vi "xmlParse.vi"() -> ()   [LabVIEW 2018]
doc: "This example demonstrates how to query an XML document by using an XPath expression and returns all the nodes that match the XPath expression."
uses:
  <vilib>/xml/Close Reference(Node).vi
  <resource>/objmgr/DOMUserDefRef.rc
  <vilib>/xml/NI_XML.lvlib
panel:
  out "concatenated string":string
  out "Array":string[](array[string])
  out "offset past replacement 2":i32
  out "result string 2":string
  out "substring before match 2":string
  out "offset past replacement":i32
  in  "Numeric":i32
  out "size(s)":i32
  out "result string":string
  out "element":string
  in  "XML File Path":path=path "C:/LabviewFiles/LabView/learning(Lee)/LVU examples/xmlParsing/ETNT22116.xml"
  out "XML":string
  in  "XPath Expression":string
  out "Search Results":string[](array[string])
  # "filter for software"
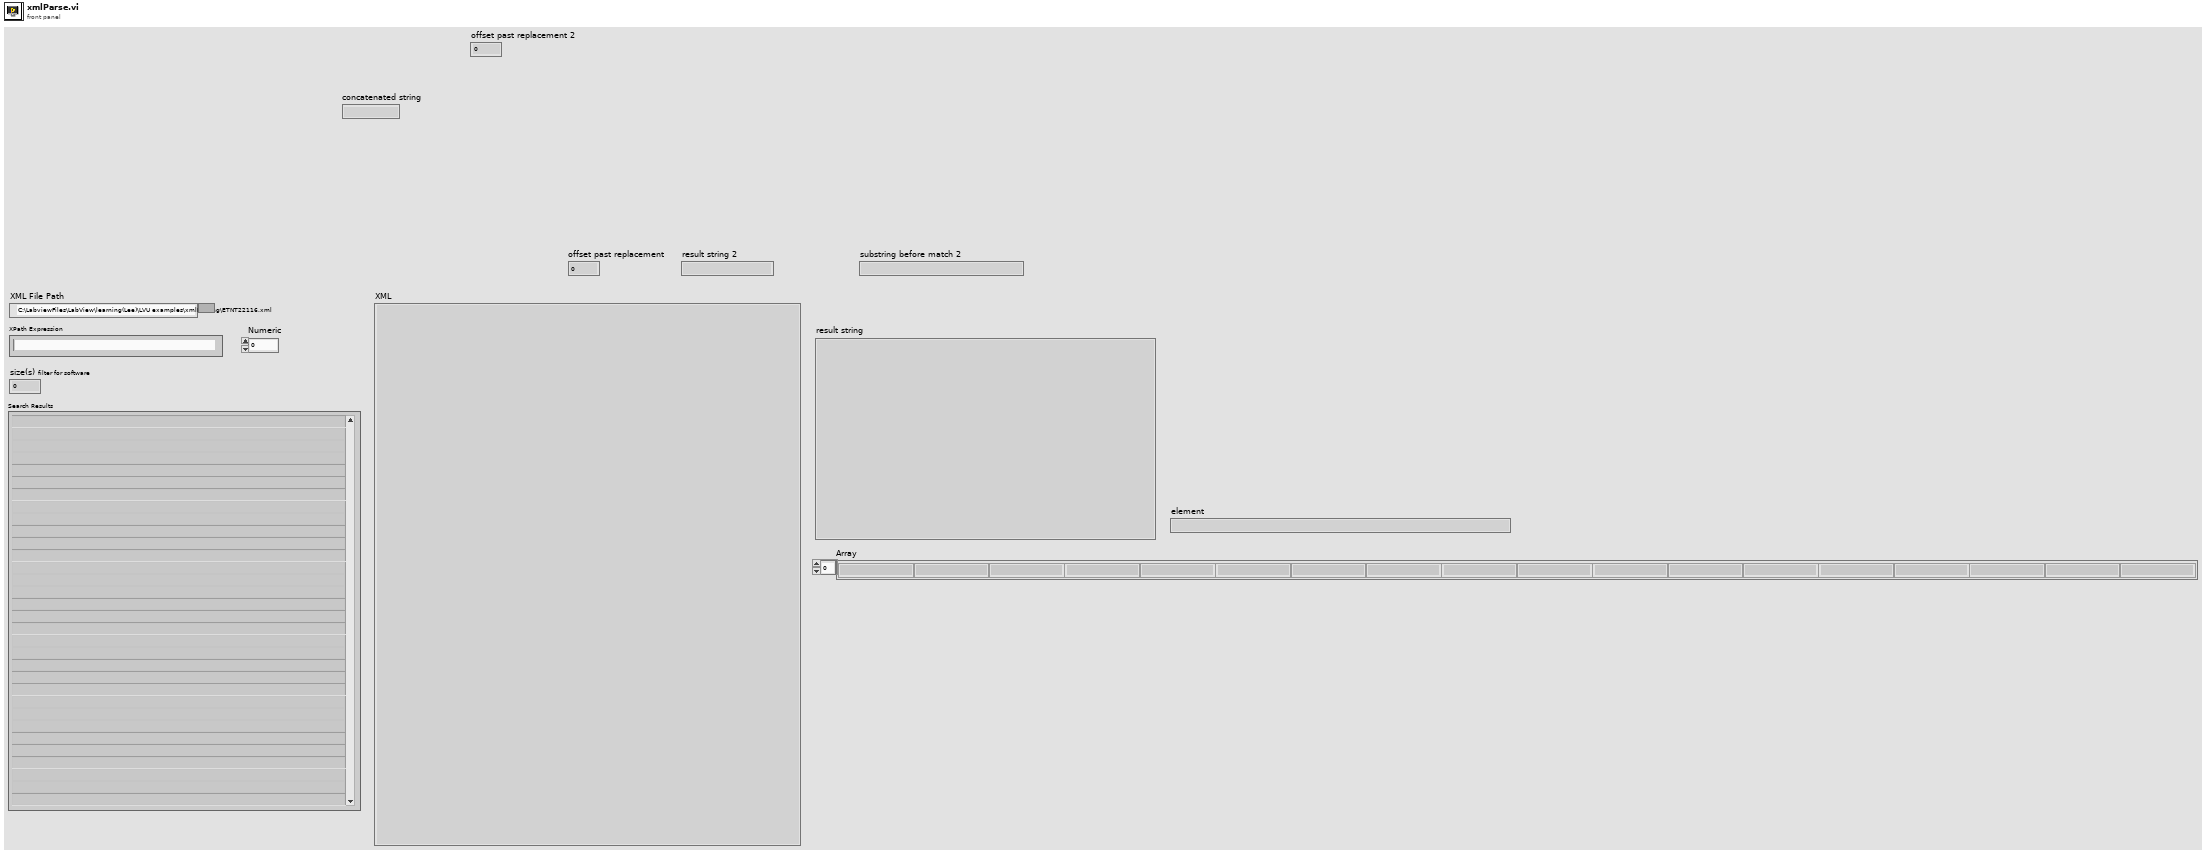
[diagram p1: front panel]
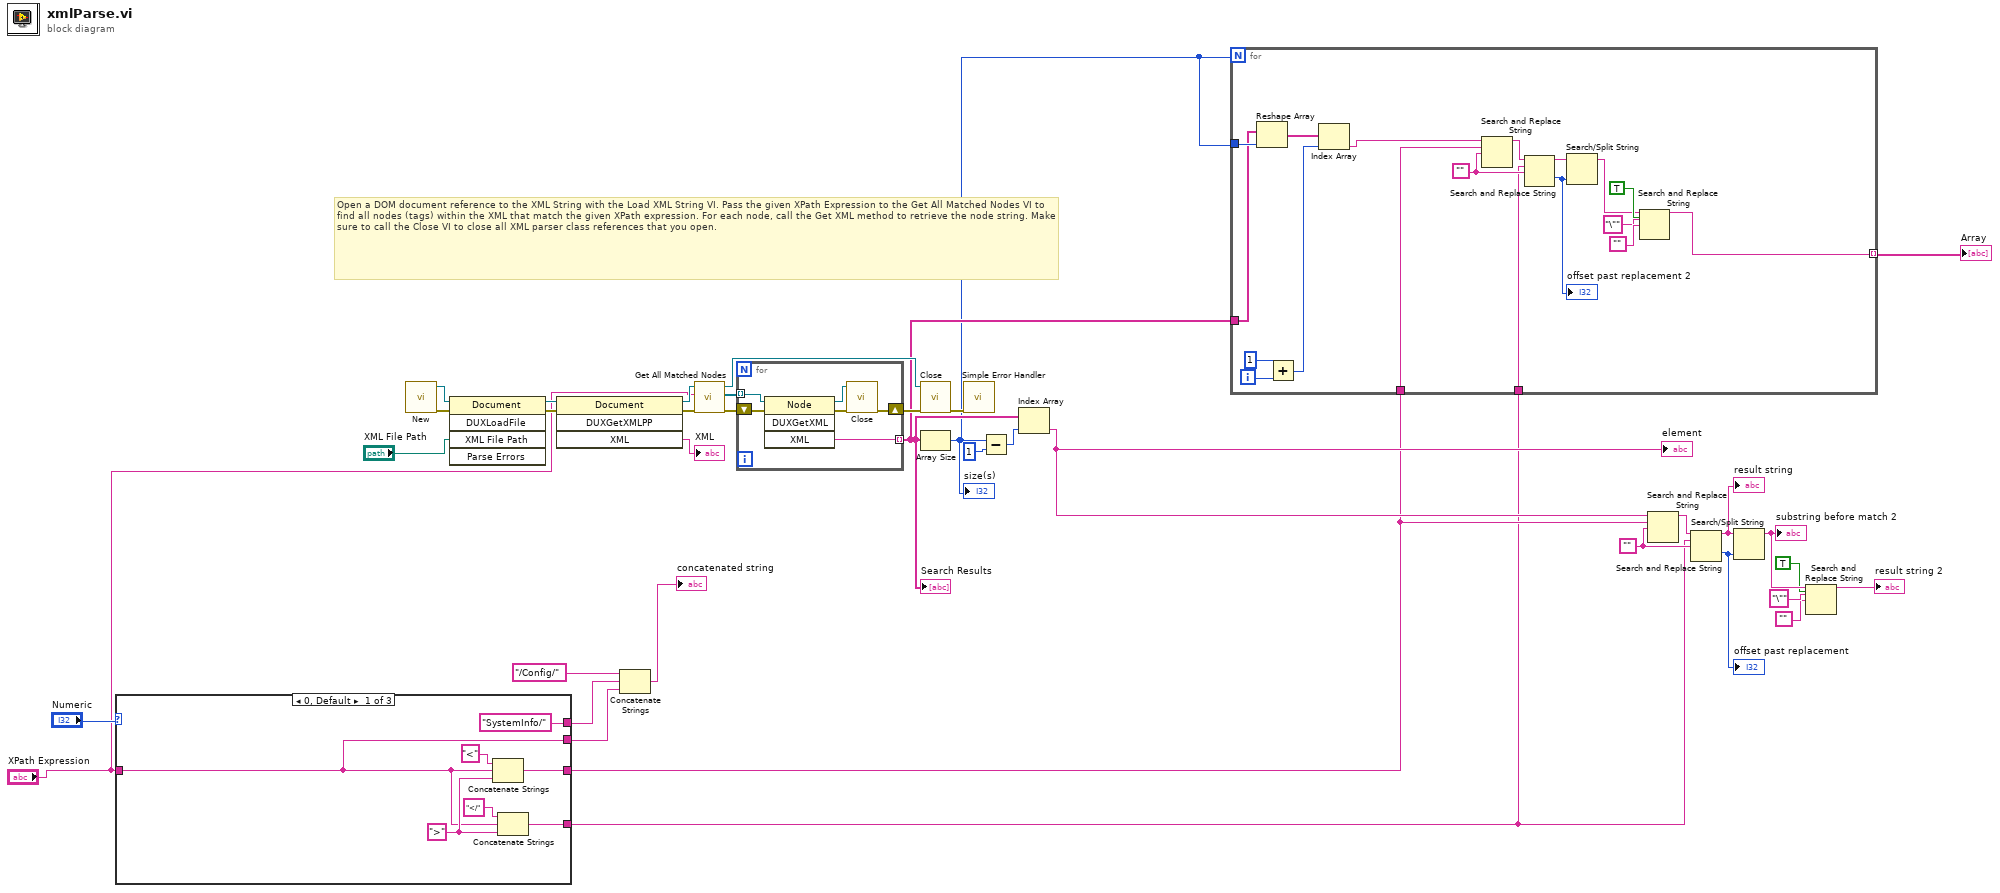
[diagram p0: block diagram]
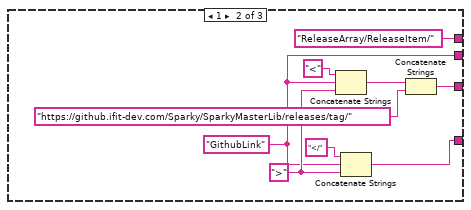
[diagram p2: hidden frame]
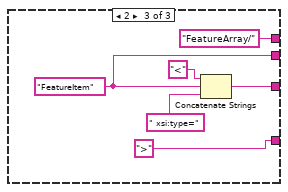
[diagram p3: hidden frame]
diagram:
  w15 = ""
  # "Open a DOM document reference to the XML String with the Load XML String VI. Pass the given XPath Expression to the Get All Matched Nodes VI to find all nodes (tags) within the XML that match the given XPath expression. For each node, call the Get XML method to retrieve the node string. Make sure to call the Close VI to close all XML parser class references that you open."
  n1 = case shown="0, Default" "Numeric" {
    tunnel: ["SystemInfo/" "ReleaseArray/ReleaseItem/" "FeatureArray/"] -> w18
    tunnel: [w39 w48 ">" ("string")] -> w4
    tunnel: [w38 w47 w56] -> w5
    tunnel: [w37 w44 w53] -> w17
    tunnel: "XPath Expression" -> [w37 _ _]
    frame 0, Default {
      w41 = ">" ("string")
      n2 = Concatenate Strings("<" ("string"), w37, w41) -> (w38:string)
      n3 = Concatenate Strings("</" ("string"), w37, w41) -> (w39:string)
    }
    frame 1 {
      w44 = "GithubLink"
      w50 = ">" ("string")
      n4 = Concatenate Strings("<" ("string"), w44, w50) -> (w46:string)
      n5 = Concatenate Strings("</" ("string"), w44, w50) -> (w48:string)
      n6 = Concatenate Strings(w46, "https://github.ifit-dev.com/Sparky/SparkyMasterLib/releases/tag/") -> (w47:string)
    }
    frame 2 {
      w53 = "FeatureItem"
      n7 = Concatenate Strings("<" ("string"), w53, " xsi:type=") -> (w56:string)
    }
  }
  n8 = call <vilib>:"New.vi"() -> ("error out"=w29:errorcluster, "DOM document out"=w28:refnum<k20>)  [unwired: 8 in]
  n9 = invoke class="Document" method="DUXLoadFile"(reference=w28, error in=w29, "XML File Path"="XML File Path") -> (reference out=w31:refnum<k20>, error out=w30:errorcluster)  [unwired: 2 in, 3 out]
  n10 = invoke class="Document" method="DUXGetXMLPP"(reference=w31, error in=w30) -> (reference out=w27:refnum<k20>, error out=w25:errorcluster, "XML"=→"XML":string)  [unwired: 2 in, 1 out]
  n11 = Concatenate Strings("/Config/" ("string"), w18, w17) -> (→"concatenated string":string)
  n12 = call <vilib>:"Get All Matched Nodes.vi"("error in (no error)"=w25, "XPath expression"="XPath Expression", "node in"=w27) -> ("error out"=w35:errorcluster, "node result array"=w36:refnum<k20>[], "node out"=w33:refnum<k20>)  [unwired: 6 out]
  n13 = for {
    tunnel: w36 -> [w60] mode=indexing
    shift-right: [w62] -> w34
    shift-left: w35 -> [w61]
    tunnel: [w59] -> w6 mode=indexing
    n14 = invoke on="Invoke Node" class="Node" method="DUXGetXML"(reference=w60, error in=w61) -> (reference out=w63:refnum<k20>, error out=w64:errorcluster, "XML"=w59:string)  [unwired: 2 in, 1 out]
    n15 = call-poly <vilib>:"Close.vi"("error in (no error)"=w64, "node"=w63) -> ("error out"=w62:errorcluster)  [unwired: 7 out]
  }
  "Search Results" <- w6
  n16 = call-poly <vilib>:"Close.vi"("error in (no error)"=w34, "node"=w33) -> ("error out"=w32:errorcluster)  [unwired: 7 out]
  n17 = Array Size(array=w6) -> (size(s)=w3:i32)
  "size(s)" <- w3
  n18 = call <vilib>:"Simple Error Handler.vi"("error in (no error)"=w32) -> ()  [unwired: 1 in, 8 out]
  n19 = Subtract(x=w3, y=1) -> (x-y=w23:i32)
  n20 = Index Array(array=w6, index=w23) -> (element=w16:string)
  "element" <- w16
  n21 = for {
    N: w3 -> [_]
    tunnel: w6 -> [w67]
    tunnel: w5 -> [w72]
    tunnel: w4 -> [w71]
    tunnel: w3 -> [w69]
    tunnel: [w68] -> w2 mode=indexing
    i -> [w82]
    w73 = ""
    n22 = Reshape Array(w67, w69) -> (w66:string[])
    n23 = Add(x=1, y=w82) -> (x+y=w70:i32)
    n24 = Index Array(array=w66, index=w70) -> (element=w65:string)
    n25 = Search and Replace String(input string=w65, search string=w72, replace string=w73) -> (result string=w74:string)  [unwired: 5 in, 3 out]
    n26 = Search and Replace String(input string=w74, search string=w71, replace string=w73) -> (result string=w76:string, offset past replacement=w75:i32)  [unwired: 5 in, 2 out]
    "offset past replacement 2" <- w75
    n27 = Search/Split String(string=w76, offset (0)=w75) -> (substring before match=w77:string)  [unwired: 1 in, 2 out]
    n28 = Search and Replace String(replace all?=TRUE ("replace all? (F)"), input string=w77, search string="\"", replace string="") -> (result string=w68:string)  [unwired: 4 in, 3 out]
  }
  "Array" <- w2
  n29 = Search and Replace String(input string=w16, search string=w5, replace string=w15) -> (result string=w14:string)  [unwired: 5 in, 3 out]
  n30 = Search and Replace String(input string=w14, search string=w4, replace string=w15) -> (result string=w12:string, offset past replacement=w13:i32)  [unwired: 5 in, 2 out]
  "result string" <- w12
  "offset past replacement" <- w13
  n31 = Search/Split String(string=w12, offset (0)=w13) -> (substring before match=w11:string)  [unwired: 1 in, 2 out]
  "substring before match 2" <- w11
  n32 = Search and Replace String(replace all?=TRUE ("replace all? (F)"), input string=w11, search string="\"", replace string="") -> (result string=→"result string 2":string)  [unwired: 4 in, 3 out]
